vi "path tag constant.vi"() -> (3 "Tag":string)   [LabVIEW 2013, in "file errors.lvlib"]
uses:
  file errors.lvlib
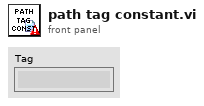
[diagram p1: front panel]
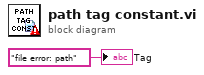
[diagram p0: block diagram]
diagram:
  "Tag" <- "file error: path" ("Tag")
